vi "SRV_ConvertToC.vi"(3 "SuperPro":T1) -> (0 "download?":bool, 1 "C":string)   [LabVIEW 2009]
uses:
  <userlib>/SuperPro/OpCodes/_SubVIs/SuperProControl.ctl
panel:
  # "This LabVIEW item is deprecated.\n\nIt is believed to be unused and will be removed in a future version of SRV."
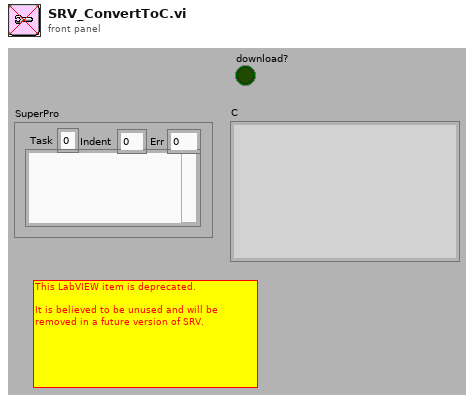
[diagram p1: front panel]
types:
  T1 = typedef "SuperProControl.ctl" = cluster{"Task":i32, "Indent":i32, "Err":i32, "ASM":string}
  T2 = cluster{"Name":string, "type":enum16{"boolean", "u8", "i8", "u16", "i16", "u32", "i32", "u64", "i64", "SGL", "DBL", "EXT", "CPX"}}[]
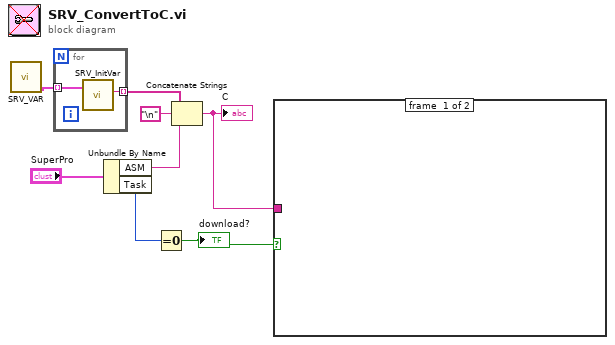
[diagram p0: block diagram]
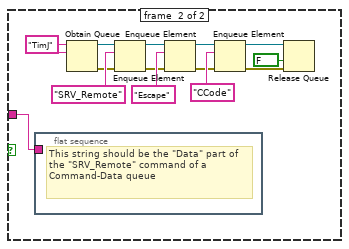
[diagram p2: hidden frame]
diagram:
  n1 = call "SRV_VAR.vi"() -> ("Variables"=w8:T2)  [unwired: 3 in, 3 out]
  n2 = for {
    tunnel: w8 -> [w10] mode=indexing
    tunnel: [w9] -> w5 mode=indexing
    n3 = call "SRV_InitVar.vi"("Variable"=w10) -> ("String"=w9:string)  [unwired: 1 in]
  }
  n4 = Unbundle By Name("SuperPro") -> ("ASM"=w6:string, "Task"=w3:i32)
  n5 = Equal To 0?(x=w3) -> (x = 0?=w2:bool)
  "download?" <- w2
  n6 = Concatenate Strings(w5, "\n", w6) -> (w1:string)
  "C" <- w1
  n7 = case shown="True" w2 {
    tunnel: w1 -> [_ w17]
    frame #0 {
    }
    frame #1 {
      w23 = "TimJ" ("name (unnamed)")
      n8 = flat-sequence {
        tunnel: w17 -> [_]
        frame #0 {
          # "This string should be the \"Data\" part of the \"SRV_Remote\" command of a Command-Data queue"
        }
      }
      n9 = Obtain Queue(name (unnamed)=w23, element data type=w23) -> (queue out=w24:refnum<queue>, error out=w16:errorcluster)  [unwired: 3 in, 1 out]
      n10 = Enqueue Element(queue=w24, element="SRV_Remote" ("name (unnamed)"), error in (no error)=w16) -> (queue out=w20:refnum<queue>, error out=w15:errorcluster)  [unwired: 1 in, 1 out]
      n11 = Enqueue Element(queue=w20, element="Escape" ("name (unnamed)"), error in (no error)=w15) -> (queue out=w19:refnum<queue>, error out=w14:errorcluster)  [unwired: 1 in, 1 out]
      n12 = Enqueue Element(queue=w19, element="CCode" ("name (unnamed)"), error in (no error)=w14) -> (queue out=w13:refnum<queue>, error out=w12:errorcluster)  [unwired: 1 in, 1 out]
      n13 = Release Queue(queue=w13, force destroy? (F)=FALSE, error in (no error)=w12) -> ()  [unwired: 3 out]
    }
  }
